vi "RT Loop - Analyze Acceleration_high_speed.vi"(3 "queue out":refnum<queue>, 7 "testing":bool, 8 "error in (no error)":errorcluster, 9 "Acceleration RT FIFO In":T1, 10 "FPGA VI Reference Out 2":refnum<k20>, 11 "Message Queue":refnum<queue>) -> (1 "Acceleration RT FIFO Out":T1)   [LabVIEW 2017]
doc: "Read and analyze acceleration waveform data from FPGA via DMA FIFO. If the acceleration is over the limit, then send the acceleration waveform data to the Log Data Loop."
uses:
  UI Error Handlers/support/Message Queue/Message Cluster.ctl
  controls/Acceleration RT FIFO Reference.ctl
  data_sav.ctl
  Control 1.ctl
  Globals/Global - All RT Loop Stop.vi
  Globals/Global - Configuration Options.vi
  <vilib>/Utility/error.llb/Error Cluster From Error Code.vi
  <vilib>/rvi/errors/niLvFpgaAdjustHostInterfaceError.vi
  <vilib>/rvi/interface/nirviMethod/nirviMethod.xnode
  <vilib>/FPGAPlugInAG/Dynamic/niLvFpga_ReadFifo_Dynamic.vi
  <vilib>/rvi/errors/niLvFpgaMergeErrorWithErrorCode.vi
  UI Error Handlers/support/Logging/Logging.lvlib
  UI Error Handlers/support/Message Queue/Message Queue.lvlib
panel:
  out "error out":errorcluster
  out "x-y":u32
  out "G1 status":cluster{"G1 trigger":bool}
  out "G1 status.G1 trigger":bool
  out "sta":bool
  out "logical OR":bool
  in  "Data Rate (Hz)":dbl
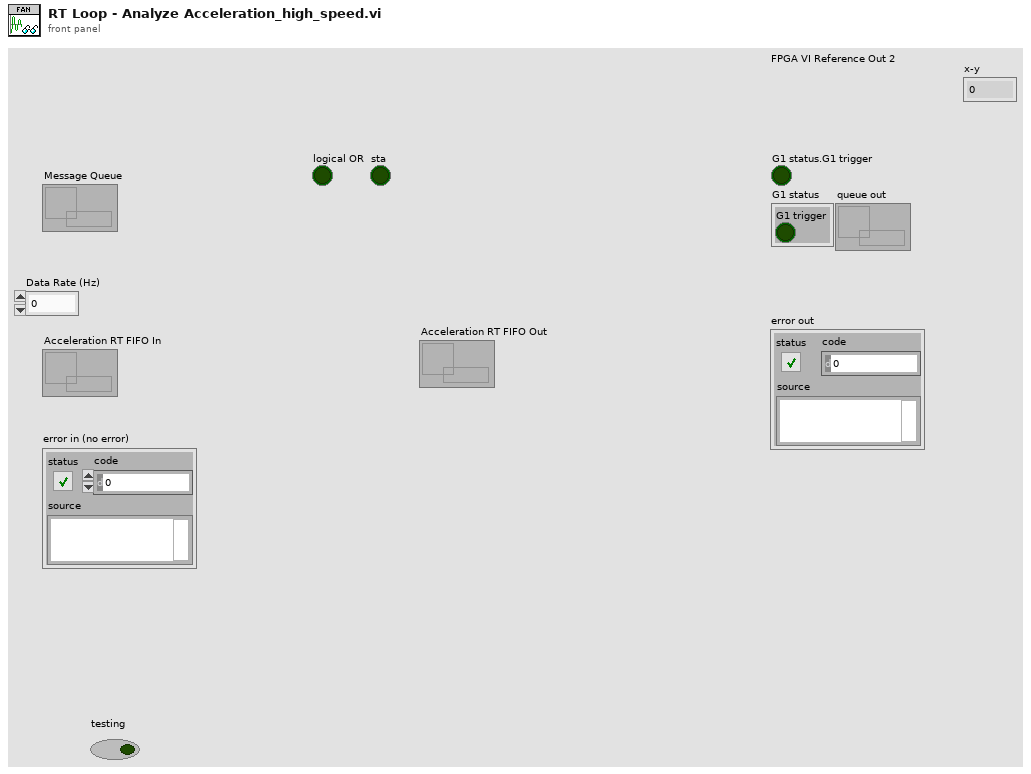
[diagram p1: front panel]
types:
  T1 = typedef "Acceleration RT FIFO Reference.ctl" = refnum<k33>
  T2 = typedef "data_sav.ctl" = cluster{"Log File out 2":refnum<k34>, "Array":T3[]}
  T3 = typedef "Control 1.ctl" = waveform(dbl)
  T4 = cluster{"Tool data":cluster{"Number of teeth":sgl}, "Cutting data":cluster{"rpm":sgl}, "Limits":cluster{"Magnitude threshold":sgl, "Tolerance":sgl}, "G1 status":cluster{"G1 trigger":bool}}
  T5 = cluster{"Log File out":refnum<k34>, waveform(dbl)[]}
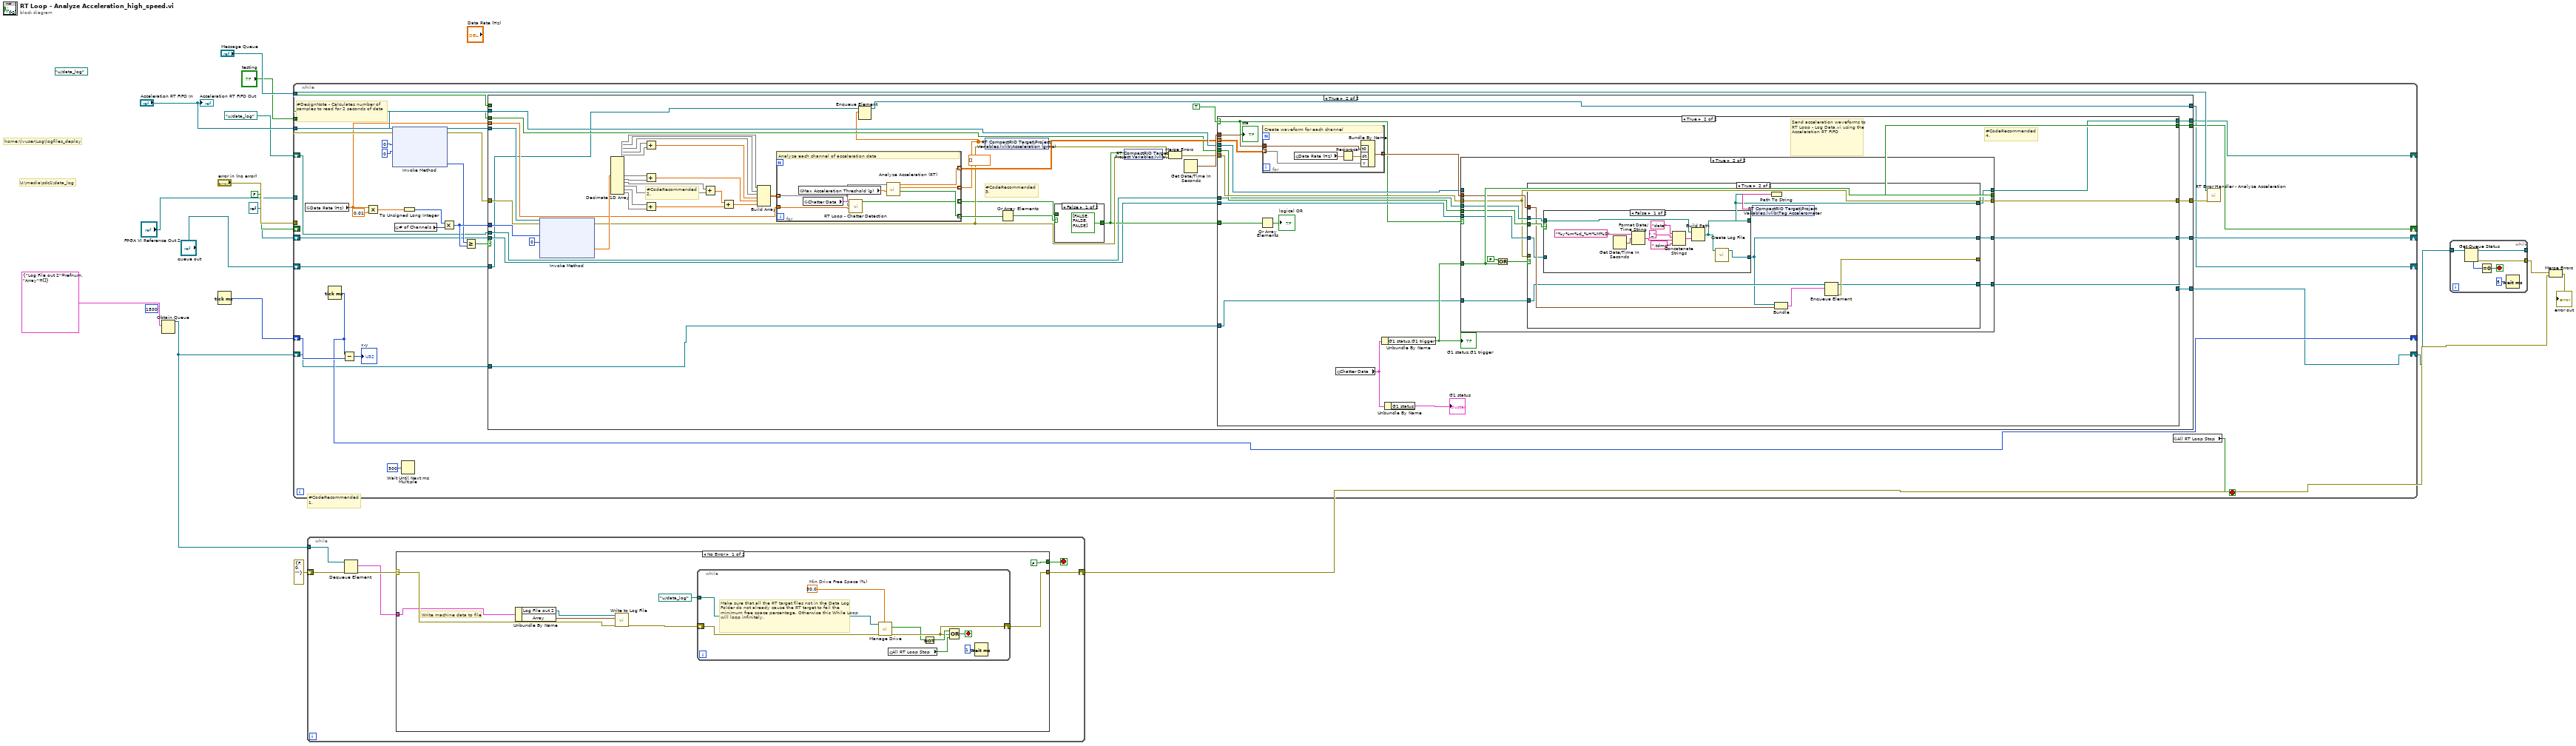
[diagram p0: block diagram]
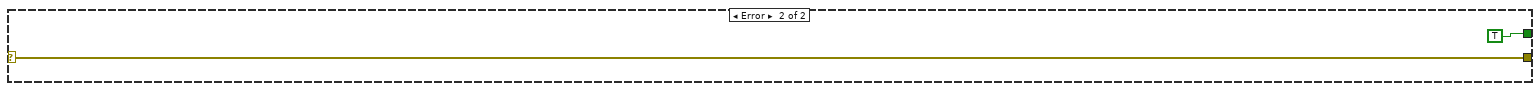
[diagram p2: hidden frame]
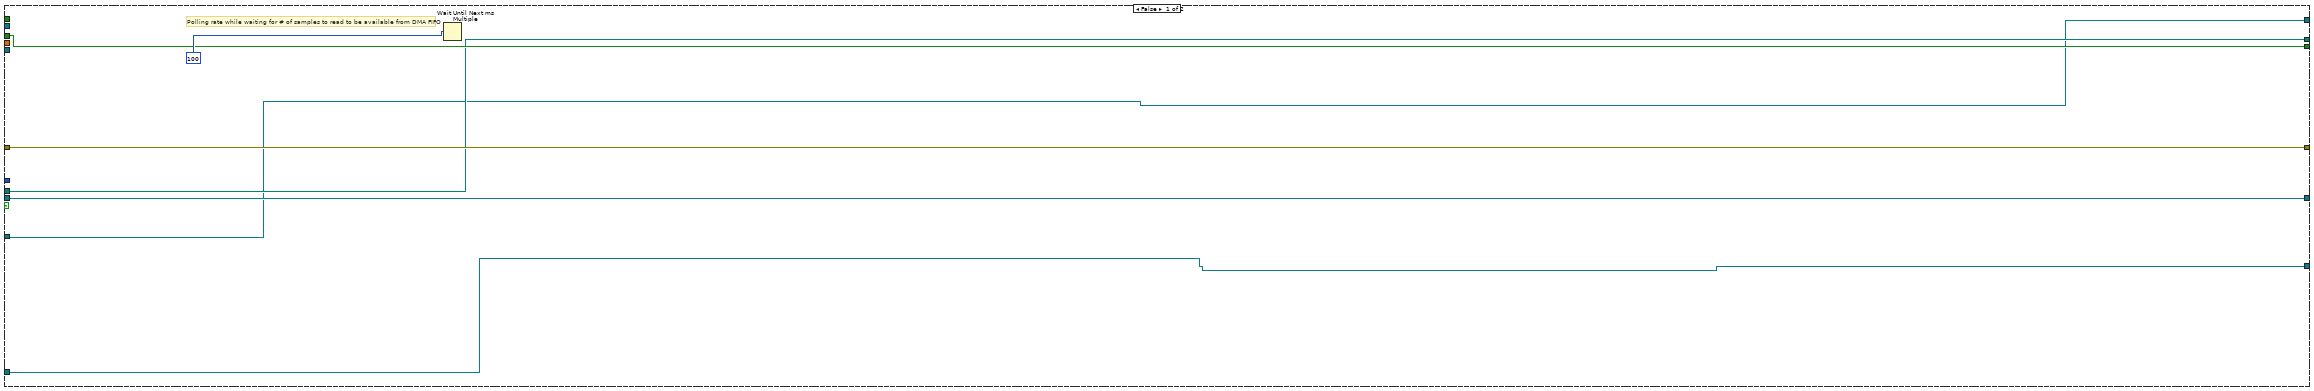
[diagram p3: hidden frame]
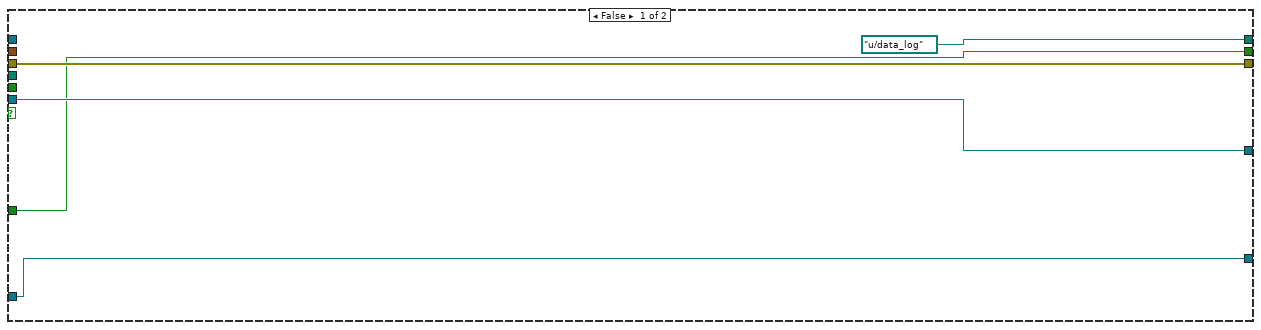
[diagram p6: hidden frame]
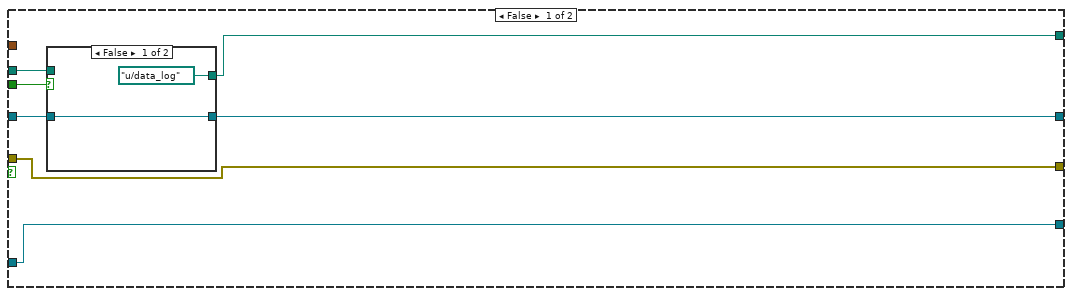
[diagram p7: hidden frame]
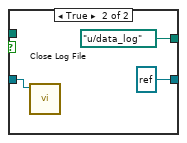
[diagram p8: hidden frame]
diagram:
  (unwired) 1500 ("max queue size (-1, unlimited)")
  (unwired) path "u:/data_log" ("AVI Path")
  # "U:\\media\\sdc1\\data_log"
  # "home:\\lvuser\\Log\\logfiles_deploy"
  # "#CodeRecommended\n1."
  n1 = Obtain Queue(element data type=T2 {"Log File out 2"=refnum, "Array"=[]}) -> (queue out=w6:refnum<queue>)  [unwired: 4 in, 2 out]
  n2 = Tick Count (ms)() -> (millisecond timer value=w10:u32)
  n3 = while {
    tunnel: "FPGA VI Reference Out 2" -> [w50]
    tunnel: "error in (no error)" -> [w49]
    tunnel: "Message Queue" -> [w42]
    tunnel: "Acceleration RT FIFO In" -> [w40]
    tunnel: "testing" -> [w32]
    shift-right: [w29] -> _
    shift-left: path "u:/data_log" ("AVI Path") -> [w28]
    shift-right: [w31] -> _
    shift-left: FALSE -> [w30]
    shift-right: [w27] -> _
    shift-left: refnum<k34> refnum ("Log File out") -> [w26]
    shift-right: [w24] -> _
    shift-left: w10 -> [w25]
    shift-right: [w20] -> _
    shift-left: "queue out" -> [w21]
    shift-right: [w19] -> w1
    shift-left: w6 -> [w22]
    stop <- w43 stop-if-true
    # "#DesignNote - Calculates number of samples to read for 2 seconds of data"
    n4 = global read "Global - Configuration Options.vi" "Data Rate (Hz)"() -> (w34:dbl)
    n5 = Tick Count (ms)() -> (millisecond timer value=w24:u32)
    n6 = Subtract(x=w24, y=w25) -> (x-y=→"x-y":u32)
    n7 = Multiply(x=w34, y=0.01) -> (x*y=w38:dbl)
    n8 = xnode "Invoke Method"("FPGA VI Reference In"=w50, "error in"=w49, "Number of Elements"=u32 0, "Timeout (ms)"=0) -> ("FPGA VI Reference Out"=w46:refnum<k20>, "error out"=w45:errorcluster, "Elements Remaining"=w33:u32)  [unwired: 1 out]
    n9 = global read "Global - Configuration Options.vi" "# of Channels"() -> (w35:u32)
    n10 = Wait Until Next ms Multiple(millisecond multiple=u32 500) -> ()  [unwired: 1 out]
    n11 = To Unsigned Long Integer(number=w38) -> (unsigned 32bit integer=w37:u32)
    n12 = Multiply(x=w37, y=w35) -> (x*y=w36:u32)
    n13 = Greater Or Equal?(x=w33, y=w36) -> (x >= y?=w44:bool)
    n14 = case shown="True" w44 {
      tunnel: w46 -> [_ w104]
      tunnel: w45 -> [w57 w103]
      tunnel: [w57 w99] -> w41
      tunnel: w36 -> [_ w102]
      tunnel: w40 -> [_ w97]
      tunnel: w34 -> [_ w94]
      tunnel: w32 -> [_ _]
      tunnel: [w55 w86] -> w31
      tunnel: w30 -> [w55 w85]
      tunnel: [w54 w84] -> w29
      tunnel: w28 -> [w54 w83]
      tunnel: [w53 w82] -> w27
      tunnel: w26 -> [w53 w81]
      tunnel: w22 -> [w52 w62]
      tunnel: [w52 w61] -> w19
      tunnel: w21 -> [w51 w60]
      tunnel: [w51 w58] -> w20
      frame False {
        # "Polling rate while waiting for # of samples to read to be available from DMA FIFO"
        n15 = Wait Until Next ms Multiple(millisecond multiple=u32 100) -> ()  [unwired: 1 out]
      }
      frame True {
        (unwired) dbl[] []
        # "#CodeRecommended\n3."
        # "#CodeRecommended\n2."
        n16 = xnode "Invoke Method"("FPGA VI Reference In"=w104, "error in"=w103, "Number of Elements"=w102, "Timeout (ms)"=0) -> ("error out"=w93:errorcluster, "Data"=w96:sgl[])  [unwired: 2 out]
        n17 = Decimate 1D Array(w96) -> (w78:sgl[], w77:sgl[], w76:sgl[], w75:sgl[], w74:sgl[], w72:sgl[], w71:sgl[], w70:sgl[], w69:sgl[], w68:sgl[], w67:sgl[])
        n18 = Add(x=w75, y=w74) -> (x+y=w73:sgl[])
        n19 = Add(x=w72, y=w71) -> (x+y=w63:sgl[])
        n20 = Add(x=w68, y=w67) -> (x+y=w65:sgl[])
        n21 = Add(x=w70, y=w69) -> (x+y=w66:sgl[])
        n22 = Add(x=w66, y=w65) -> (x+y=w64:sgl[])
        n23 = Build Array(w78, w77, w76, w73, w63, w64) -> (w79:sgl[][])
        n24 = for {
          tunnel: [w114] -> w98 mode=indexing
          tunnel: [w113] -> w95 mode=indexing
          tunnel: [w112] -> w59 mode=indexing
          tunnel: w94 -> [w110]
          tunnel: [w109] -> w88 mode=indexing
          tunnel: w79 -> [w107] mode=indexing
          # "Analyze each channel of acceleration data"
          n25 = global read "Global - Configuration Options.vi" "Max Acceleration Threshold (g)"() -> (w111:sgl)
          n26 = global read "Global - Configuration Options.vi" "Chatter Data"() -> (w108:T4)
          n27 = call "RT Loop - Chatter Detection.vi"("Data Rate (Hz)"=w110, "Acceleration Waveform (SGL)"=w107, "Chatter Data"=w108) -> ("Chatter?"=w109:bool)  [unwired: 8 in]
          n28 = call "Analyze Acceleration (RT).vi"("Max Instantaneous Acceleration (g)"=w111, "Acceleration Waveform (SGL)"=w107) -> ("Over Limit?"=w114:bool, "Acceleration (grms)"=w112:dbl, "Acceleration Waveform (DBL)"=w113:dbl[])  [unwired: 7 in]
        }
        n29 = Enqueue Element(queue=w60, element=w59) -> (queue out=w58:refnum<queue>)  [unwired: 2 in, 2 out]
        n30 = shared-variable "RT CompactRIO Target\\Project Variables.lvlib\\Acceleration (grms)"(w59, error in=w93) -> (error out=w91:errorcluster)
        n31 = Or Array Elements(Boolean array=w98) -> (logical OR=w89:bool)
        n32 = case shown="False" w89 {
          tunnel: w88 -> [_ w106]
          tunnel: [bool[] [FALSE, FALSE, FALSE] ("Chatter?") w106] -> w87
          frame False {
          }
          frame True {
          }
        }
        n33 = shared-variable "RT CompactRIO Target\\Project Variables.lvlib\\Chatter?"(w87, error in=w93) -> (error out=w92:errorcluster)
        n34 = Merge Errors(w91, w92) -> (w90:errorcluster)
        n35 = Get Date/Time In Seconds() -> (seconds since 1Jan1904=w100:timestamp)
        n36 = case shown="True" TRUE {
          selector: TRUE -> [_ w120]
          tunnel: w100 -> [_ w139]
          tunnel: w90 -> [w119 w138]
          tunnel: [w119 w123] -> w99
          tunnel: w97 -> [_ w136]
          tunnel: w95 -> [_ w135]
          tunnel: w87 -> [_ w133]
          tunnel: [w118 w130] -> w86
          tunnel: w85 -> [w118 w129]
          tunnel: [w117 w128] -> w84
          tunnel: w83 -> [w117 w124]
          tunnel: [w116 w127] -> w82
          tunnel: w81 -> [w116 w126]
          tunnel: w62 -> [w115 w122]
          tunnel: [w115 w121] -> w61
          frame False {
          }
          frame True {
            # "#CodeRecommended\n4."
            # "Send acceleration waveforms to RT Loop - Log Data.vi using the Acceleration RT FIFO"
            n37 = Or Array Elements(Boolean array=w133) -> (logical OR=→"logical OR":bool)
            n38 = for {
              tunnel: w135 -> [w196] mode=indexing
              tunnel: w139 -> [w195]
              tunnel: [w193] -> w137 mode=indexing
              # "Create waveform for each channel"
              n39 = global read "Global - Configuration Options.vi" "Data Rate (Hz)"() -> (w192:dbl)
              n40 = Reciprocal(x=w192) -> (1/x=w194:dbl)
              n41 = Bundle By Name("t0"=w195, "dt"=w194, "Y"=w196) -> (w193:waveform(dbl))  [unwired: 1 in]
            }
            n42 = global read "Global - Configuration Options.vi" "Chatter Data"() -> (w132:T4)
            n43 = Unbundle By Name(w132) -> ("G1 status.G1 trigger"=w125:bool)
            "G1 status.G1 trigger" <- w125
            n44 = Unbundle By Name(w132) -> ("G1 status"=→"G1 status":cluster{"G1 trigger":bool})
            n45 = case shown="True" w120 {
              tunnel: w138 -> [w144 w147]
              tunnel: w137 -> [_ w148]
              tunnel: w136 -> [_ _]
              tunnel: w125 -> [w142 w154]
              tunnel: [w142 w154] -> w130
              tunnel: w129 -> [_ w153]
              tunnel: [path "u:/data_log" ("AVI Path") w152] -> w128
              tunnel: w124 -> [_ w151]
              tunnel: [w143 w150] -> w127
              tunnel: w126 -> [w143 w149]
              tunnel: [w144 w147] -> w123
              tunnel: w122 -> [w140 w145]
              tunnel: [w140 w146] -> w121
              frame False {
              }
              frame True {
                n46 = Or(x=FALSE, y=w154) -> (x .or. y?=w156:bool)
                n47 = case shown="True" w156 {
                  tunnel: w151 -> [w160 w179]
                  tunnel: [w163 w176] -> w152
                  tunnel: w153 -> [w161 w178]
                  tunnel: w149 -> [w162 w170]
                  tunnel: w148 -> [_ w172]
                  tunnel: [w159 w169] -> w150
                  tunnel: w147 -> [w158 _]
                  tunnel: [w158 w175] -> _
                  tunnel: w145 -> [w157 w171]
                  tunnel: [w157 w174] -> w146
                  frame False {
                    n48 = case shown="False" w161 {
                      tunnel: [path "u:/data_log" ("AVI Path") path "u:/data_log" ("AVI Path")] -> w163
                      tunnel: w162 -> [w164 w167]
                      tunnel: w160 -> [_ _]
                      tunnel: [w164 refnum<k34> refnum ("Log File out")] -> w159
                      frame False {
                      }
                      frame True {
                        n49 = call "Close Log File.vi"("tdms file"=w167) -> ()  [unwired: 10 in, 1 out]
                      }
                    }
                  }
                  frame True {
                    n50 = case shown="False" w178 {
                      tunnel: w179 -> [w182 w191]
                      tunnel: [w181 w191] -> w176
                      tunnel: [w180 w190] -> w169
                      tunnel: w170 -> [_ w190]
                      frame False {
                        n51 = Get Date/Time In Seconds() -> (seconds since 1Jan1904=w185:timestamp)
                        n52 = Format Date/Time String(time format string (%c)="%y%m%d_%H%M%S", seconds (now)=w185) -> (date/time string=w188:string)  [unwired: 1 out]
                        n53 = Concatenate Strings("data" ("string"), "_" ("string"), w188, ".tdms" ("string")) -> (w183:string)
                        n54 = Build Path(base path=w182, name or relative path=w183) -> (appended path=w181:path)
                        n55 = call "Create Log File.vi"("Acceleration Exceeded Log Folder"=w181) -> ("Log File out"=w180:refnum<k34>)  [unwired: 9 in, 1 out]
                      }
                      frame True {
                      }
                    }
                    n56 = Path To String(path=w176) -> (string=w177:string)
                    n57 = shared-variable "RT CompactRIO Target\\Project Variables.lvlib\\Tag Accelerometer"(w177) -> ()  [unwired: 1 in, 1 out]
                    n58 = Bundle("Log File out"=w169, w172) -> (w173:T5)  [unwired: 1 in]
                    n59 = Enqueue Element(queue=w171, element=w173) -> (queue out=w174:refnum<queue>, error out=w175:errorcluster)  [unwired: 2 in, 1 out]
                  }
                }
              }
            }
            "sta" <- w120
          }
        }
      }
    }
    n60 = global read "Global - All RT Loop Stop.vi" "All RT Loop Stop"() -> (w43:bool)
    n61 = call "RT Error Handler - Analyze Acceleration.vi"("error in (no error)"=w41, "Message Queue"=w42) -> ()  [unwired: 9 in, 1 out]
  }
  n62 = while {
    tunnel: w6 -> [w197]
    shift-right: [w199] -> w5
    shift-left: errorcluster {"status"=FALSE, "code"=0, "source"=""} ("error IO") -> [w202]
    stop <- w200 stop-if-true
    n63 = Dequeue Element(queue=w197, error in (no error)=w202) -> (element=w198:T2, error out=w201:errorcluster)  [unwired: 1 in, 2 out]
    n64 = case shown="No Error" w201 {
      selector: w201 -> [w206 w220]
      tunnel: [FALSE TRUE] -> w200
      tunnel: [w208 w220] -> w199
      tunnel: w198 -> [w205 _]
      frame No Error {
        # "Write machine data to file"
        n65 = Unbundle By Name(w205) -> ("Log File out 2"=w204:refnum<k34>, "Array"=w203:T3[])
        n66 = call "Write to Log File.vi"("error in (no error)"=w206, "Array of Waveforms"=w203, "Log File in"=w204) -> ("error out"=w207:errorcluster)  [unwired: 7 in, 1 out]
        n67 = while {
          shift-right: [w214] -> w208
          shift-left: w207 -> [w215]
          tunnel: path "u:/data_log" ("AVI Path") -> [w212]
          stop <- w219 stop-if-true
          w213 = 30.0  # Min Drive Free Space (%)
          # "Make sure that all the RT target files not in the Data Log Folder do not already cause the RT target to fail the minimum free space percentage. Otherwise this While Loop will loop infinitely."
          n68 = call "Manage Drive.vi"("Min Drive Free Space (%)"=w213, "error in"=w215, "Data Folder"=w212) -> ("error out"=w214:errorcluster, "Drive Space Below Limit"=w211:bool)  [unwired: 7 in]
          n69 = global read "Global - All RT Loop Stop.vi" "All RT Loop Stop"() -> (w216:bool)
          n70 = Not(x=w211) -> (.not. x?=w218:bool)
          n71 = Compound Arithmetic op=OR(w218, w214, w216) -> (w219:bool)
          n72 = Wait (ms)(milliseconds to wait=u32 1) -> ()  [unwired: 1 out]
        }
      }
      frame Error {
      }
    }
  }
  n73 = while {
    tunnel: [w226] -> w8
    tunnel: [w224] -> _
    tunnel: w1 -> [w222]
    stop <- w225 stop-if-true
    n74 = Get Queue Status(queue=w222) -> (queue out=w224:refnum<queue>, error out=w226:errorcluster, # elements in queue=w223:i32)  [unwired: 2 in, 5 out]
    n75 = Equal To 0?(x=w223) -> (x = 0?=w225:bool)
    n76 = Wait (ms)(milliseconds to wait=u32 5) -> ()  [unwired: 1 out]
  }
  n77 = Merge Errors(w8, w5) -> (→"error out":errorcluster)
  "Acceleration RT FIFO Out" <- "Acceleration RT FIFO In"
